vi "DuraFET_Input&Output.vi"(6 "Temp Voltage":dbl[](array[numeric]), 7 "Write ro Spreadsheet?":bool, 8 "DirecTemp":dbl=23.4, 9 "pH voltage":dbl[](array[numeric]), 10 "Sensor in":string(combo)="MSFET 208", 11 "Spec. On Front Panel":path=path "C:/Users/Garrett/Google Drive/Documents/Martz Lab/LabView/pH_Voltages.csv") -> (0 "DuraFET Temp":dbl, 1 "Mean5":dbl=nan format="%.5f", 2 "std5":dbl=nan format="%.5f", 3 "pH voltage mean":dbl=0.012122367612086788 format="%.5f", 4 "pH voltage stdev":dbl=0.002814230140480331 format="%.5f", 5 "pHint":dbl=39.163636363636364)   [LabVIEW 2018]
uses:
  <vilib>/Utility/file.llb/Write Delimited Spreadsheet (string).vi
  <vilib>/Analysis/NI_AALBase.lvlib
  <vilib>/ptbypt/NI_PtbyPt.lvlib
panel:
  out "standard deviation":dbl format="%0.2f"
  out "5 minutes chart for pH voltage":dbl(graph)
  # "Temperature"
  # "Directemp"
  # "Durafet"
  # "pH stuff"
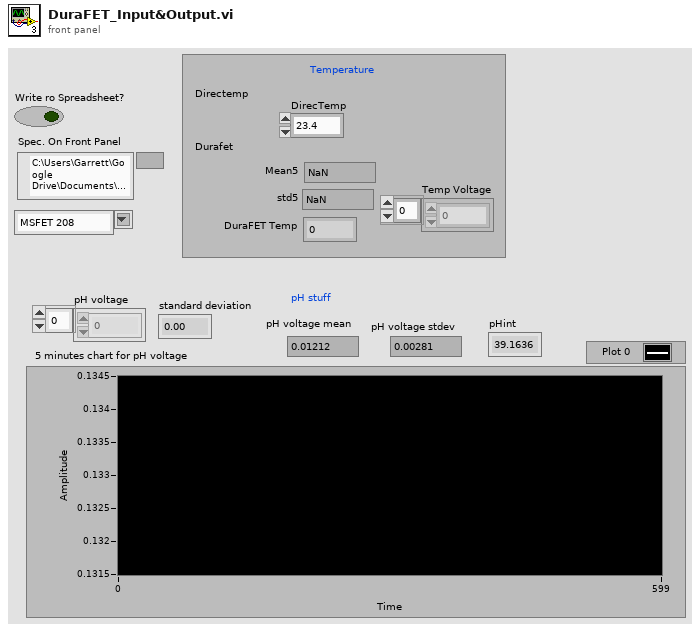
[diagram p1: front panel]
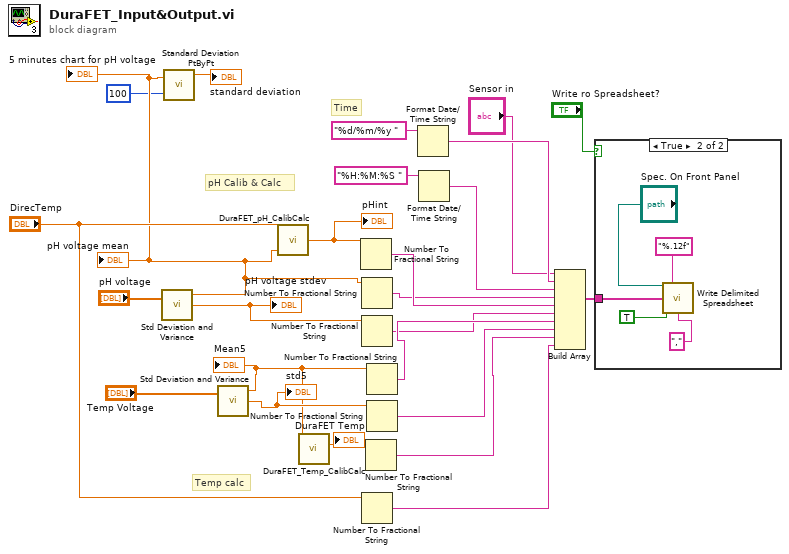
[diagram p0: block diagram]
diagram:
  # "Time"
  # "Temp calc"
  # "pH Calib & Calc"
  n1 = call <vilib>:"Std Deviation and Variance.vi"("X"="pH voltage") -> ("mean"=w3:dbl, "standard deviation"=w17:dbl)  [unwired: 1 in, 1 out]
  "pH voltage mean" <- w3
  "pH voltage stdev" <- w17
  "5 minutes chart for pH voltage" <- w3
  n2 = call <vilib>:"Standard Deviation PtByPt.vi"("x"=w3, "sample length"=100) -> ("standard deviation"=→"standard deviation":dbl)  [unwired: 1 in, 2 out]
  n3 = call <vilib>:"Std Deviation and Variance.vi"("X"="Temp Voltage") -> ("mean"=w9:dbl, "standard deviation"=w16:dbl)  [unwired: 1 in, 1 out]
  "Mean5" <- w9
  "std5" <- w16
  n4 = call "DuraFET_pH_CalibCalc.vi"("Eint: (mean voltage)"=w3, "Directemp (C)"="DirecTemp") -> ("pHint_tot"=w10:dbl)  [unwired: 1 in]
  "pHint" <- w10
  n5 = call "DuraFET_Temp_CalibCalc.vi"("Voltage from Thermistor"=w9) -> ("Temperature (C)"=w8:dbl)  [unwired: 9 in, 1 out]
  "DuraFET Temp" <- w8
  n6 = Number To Fractional String(number=w10) -> (F-format string=w15:string)  [unwired: 3 in]
  n7 = Number To Fractional String(number=w3) -> (F-format string=w11:string)  [unwired: 3 in]
  n8 = Number To Fractional String(number=w17) -> (F-format string=w18:string)  [unwired: 3 in]
  n9 = Number To Fractional String(number="DirecTemp") -> (F-format string=w7:string)  [unwired: 3 in]
  n10 = Number To Fractional String(number=w8) -> (F-format string=w22:string)  [unwired: 3 in]
  n11 = Number To Fractional String(number=w9) -> (F-format string=w20:string)  [unwired: 3 in]
  n12 = Number To Fractional String(number=w16) -> (F-format string=w21:string)  [unwired: 3 in]
  n13 = Format Date/Time String(time format string (%c)="%d/%m/%y ") -> (date/time string=w24:string)  [unwired: 2 in]
  n14 = Format Date/Time String(time format string (%c)="%H:%M:%S ") -> (date/time string=w25:string)  [unwired: 2 in]
  n15 = Build Array("Sensor in", w24, w25, w11, w15, w18, w20, w21, w22, w7) -> (w12:string[])
  n16 = case shown="True" "Write ro Spreadsheet?" {
    tunnel: w12 -> [_ w26]
    frame False {
    }
    frame True {
      n17 = call-poly <vilib>:"Write Delimited Spreadsheet.vi"("file path (dialog if empty)"="Spec. On Front Panel", "format (%s)"="%.12f" ("format (%.3f)"), "1D data"=w26, "append to file? (new file:F)"=TRUE, "delimiter (\\t)"="," ("delimiter (\\t)")) -> ()  [unwired: 9 in, 2 out]
    }
  }
